vi "comparing strings.vi"() -> ()   [LabVIEW 2018]
panel:
  out "String 2":string
  in  "String":string
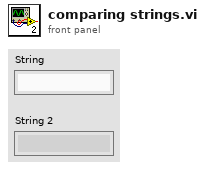
[diagram p1: front panel]
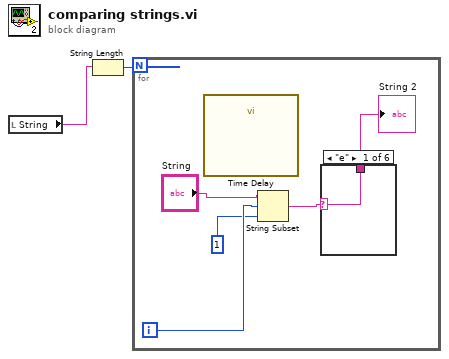
[diagram p0: block diagram]
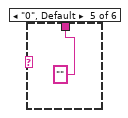
[diagram p5: hidden frame]
diagram:
  n1 = local read "String"() -> (w2:string)
  n2 = String Length(string=w2) -> (length=w1:i32)
  n3 = for {
    N: w1 -> [_]
    i -> [w7]
    n4 = call "Time Delay"() -> ()  [unwired: 11 in, 1 out]
    n5 = String Subset(string="String", offset (0)=w7, length (rest)=1 ("length (rest)")) -> (substring=w5:string)
    n6 = case shown="\"e\"" w5 {
      selector: w5 -> [w8 w9 w10 w11 _ w13]
      tunnel: [w8 w9 w10 w11 "" w13] -> w4
      frame "e" {
      }
      frame "i" {
      }
      frame "o" {
      }
      frame "u" {
      }
      frame "0", Default {
      }
      frame "a" {
      }
    }
    "String 2" <- w4
  }
